vi "test2DArray.vi"() -> (0 "error out":errorcluster)   [LabVIEW 2017, in "Assertion.Tests.lvlib" / "AssertCount.lvlib"]
uses:
  AssertCount.lvlib
  Assertion/Assertion.lvlib
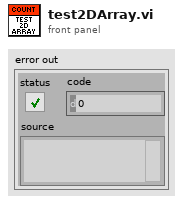
[diagram p1: front panel]
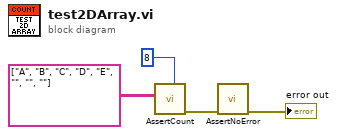
[diagram p0: block diagram]
diagram:
  n1 = call "AssertCount.vi"("Expected"=8, "Haystack"=string[][] [["A", "B", "C", "D"], ["E", "", "", ""]]) -> ("error out"=w2:errorcluster)  [unwired: 9 in]
  n2 = call "AssertNoError.vi"("error in (no error)"=w2) -> ("error out"=→"error out":errorcluster)  [unwired: 10 in]
